vi "Contour_Automatic.vi"(4 "Properties":T2={"Label Contours"=FALSE, "Line"={"Style"=enum."Automatic", "Color"=2147483647, "Width"=nan}, "Display"={"Alpha"=nan, "Z Order"=nan}} {"Line"."Color" items=["Automatic"=2147483647, "Black"=0, "White"=16777215, "Red"=16711680, "Green"=2263842, "Blue"=255, "Cyan"=65535, "Magenta"=16711935, "Yellow"=16776960]}, 5 "Levels":i32=-1, 6 "Contour Range":T1={"Min Level"=nan, "Max Level"=nan}, 7 "Z Data":dbl[][](array[numeric]), 8 "error in (no error)":errorcluster, 9 "Y Coordinates":dbl[](array[numeric]), 10 "X Coordinates":dbl[](array[numeric]), 11 "Plot ID":T7 format="%x") -> (0 "error out":errorcluster, 3 "Plot ID Out":T7 format="%x")   [LabVIEW 2013, in "Advanced Plotting Toolkit.lvlib"]
doc: "Make a 2D contour plot, with a specific number of evenly-spaced contour lines."
uses:
  Advanced Plotting Toolkit.lvlib
  typedefs/PlotID.ctl
  ContourProperties.ctl
  properties/Line.ctl
  properties/Line_Style.ctl
  typedefs/PlotColor.ctl
  properties/Display.ctl
  ContourRange.ctl
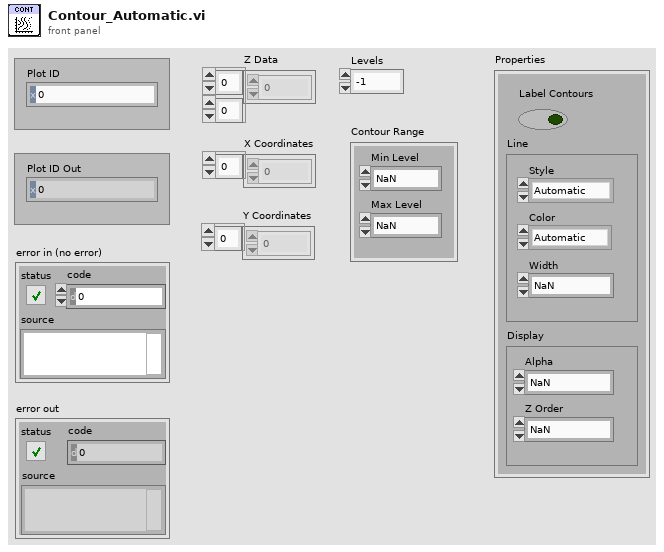
[diagram p1: front panel]
types:
  T1 = typedef "Advanced Plotting Toolkit.lvlib/ContourRange.ctl" = cluster{"Min Level":dbl, "Max Level":dbl}
  T2 = typedef "Advanced Plotting Toolkit.lvlib/ContourProperties.ctl" = cluster{"Label Contours":bool, "Line":T3, "Display":T6}
  T3 = typedef "Advanced Plotting Toolkit.lvlib/Line.ctl" = cluster{"Style":T4, "Color":T5, "Width":sgl}
  T4 = typedef "Advanced Plotting Toolkit.lvlib/Line_Style.ctl" = enum16{"Automatic", "Solid", "Dashed", "Dotted", "Dash-dot", "Invisible"}
  T5 = typedef "Advanced Plotting Toolkit.lvlib/PlotColor.ctl" = u32
  T6 = typedef "Advanced Plotting Toolkit.lvlib/Display.ctl" = cluster{"Alpha":dbl, "Z Order":dbl}
  T7 = typedef "Advanced Plotting Toolkit.lvlib/PlotID.ctl" = i32
  T8 = typedef "Advanced Plotting Toolkit.lvlib/KeyValue.ctl" = cluster{"Key":string, "Value":string}
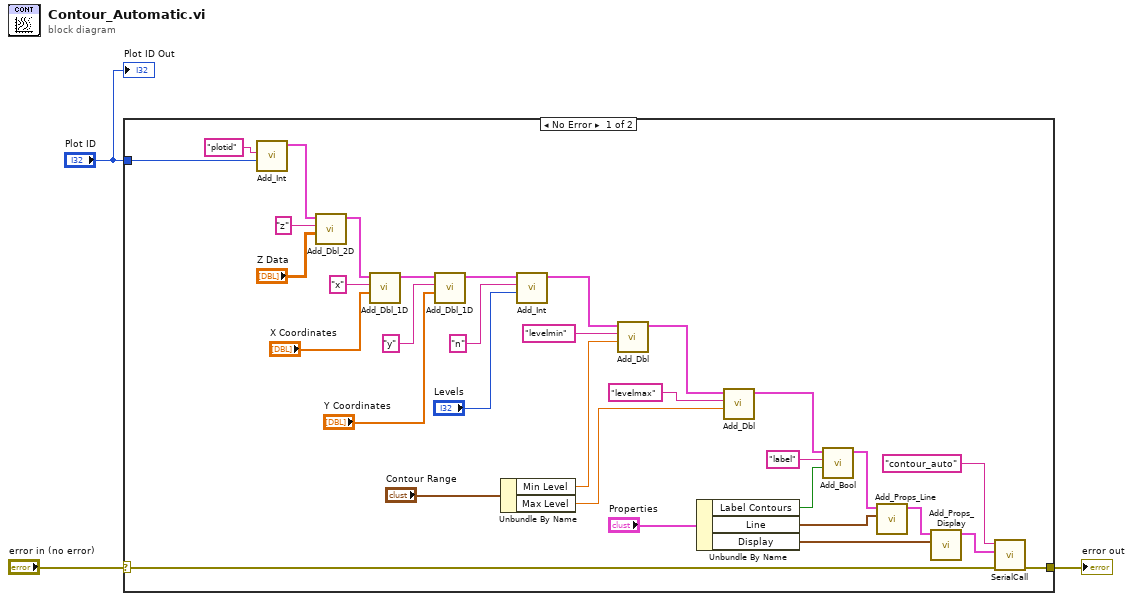
[diagram p0: block diagram]
diagram:
  n1 = case shown="No Error" "error in (no error)" {
    selector: "error in (no error)" -> [w24 w37]
    tunnel: "Plot ID" -> [w22 _]
    tunnel: [w23 w37] -> w1
    frame No Error {
      n2 = call "Add_Int.vi"("Value"=w22, "Key"="plotid") -> ("Keyword Array Out"=w31:T8[])  [unwired: 9 in]
      n3 = call "Add_Dbl_2D.vi"("Value"="Z Data", "Key"="z", "Keyword Array"=w31) -> ("Keyword Array Out"=w30:T8[])  [unwired: 8 in]
      n4 = call "Add_Dbl_1D.vi"("Value"="X Coordinates", "Key"="x", "Keyword Array"=w30) -> ("Keyword Array Out"=w29:T8[])  [unwired: 8 in]
      n5 = call "Add_Dbl_1D.vi"("Value"="Y Coordinates", "Key"="y", "Keyword Array"=w29) -> ("Keyword Array Out"=w28:T8[])  [unwired: 8 in]
      n6 = Unbundle By Name("Contour Range") -> ("Min Level"=w10:dbl, "Max Level"=w8:dbl)
      n7 = call "Add_Int.vi"("Value"="Levels", "Key"="n", "Keyword Array"=w28) -> ("Keyword Array Out"=w7:T8[])  [unwired: 8 in]
      n8 = call "Add_Dbl.vi"("Value"=w10, "Key"="levelmin", "Keyword Array"=w7) -> ("Keyword Array Out"=w6:T8[])  [unwired: 8 in]
      n9 = Unbundle By Name("Properties") -> ("Label Contours"=w14:bool, "Line"=w16:T3, "Display"=w15:T6)
      n10 = call "Add_Dbl.vi"("Value"=w8, "Key"="levelmax", "Keyword Array"=w6) -> ("Keyword Array Out"=w5:T8[])  [unwired: 8 in]
      n11 = call "Add_Bool.vi"("Value"=w14, "Key"="label", "Keyword Array"=w5) -> ("Keyword Array Out"=w13:T8[])  [unwired: 8 in]
      n12 = call "Add_Props_Line.vi"("Line"=w16, "Keyword Array"=w13) -> ("Keyword Array Out"=w4:T8[])  [unwired: 9 in]
      n13 = call "Add_Props_Display.vi"("Display"=w15, "Keyword Array"=w4) -> ("Keyword Array Out"=w17:T8[])  [unwired: 9 in]
      n14 = call "SerialCall.vi"("error in (no error)"=w24, "data"=w17, "Resource"="contour_auto") -> ("error out"=w23:errorcluster)  [unwired: 7 in, 1 out]
    }
    frame Error {
    }
  }
  "error out" <- w1
  "Plot ID Out" <- "Plot ID"
